vi "Read GMLAN PIDs and DTCs.vi"(8 "error in (no error)":errorcluster, 11 "State Variables":T1={"TCP Refs"={"Connection List"=refnum, "listener ID"=refnum}, "Stop"=refnum, "Top VI"=refnum, "Parameters"={"Name"="", "PID Lookup"=variant, "DID Lookup"=variant, "Section Properties"={"CAN"={"Database File"=path "", "CAN Interface"=enum."CAN0", "Baud Rate"=0, "Diagnostic Protocol"=enum."GMLAN", "Transport Protocol"=enum."ISO TP - Normal Mode", "Transmit ID"=0, "Receive ID"=0, "Transmit Extension"=0, "Receive Extension"=0, "Receive UUDT ID"=0, "Enable Stream"=TRUE, "VW TP Channel ID"=0}, "DPIDs"=[], "DTC descriptor"={"DTC Byte Length"=2, "Status Byte Length"=1, "Add Data Byte Length"=1, "Byte Order"=enum."Motorola"}, "PIDs"=[], "DIDs"=[], "CPIDs"=[]}, "ChanRefs"={"ToVS.PIDs"={"Name"="", "Write to VS Engine FIFO"=refnum, "Pairs"={"Refs"=[], "Values"=[]}}, "ToVS.DIDs"={"Name"="", "Write to VS Engine FIFO"=refnum, "Pairs"={"Refs"=[], "Values"=[]}}, "ToVS.DTCs"={"Name"="", "Write to VS Engine FIFO"=refnum, "Pairs"={"Refs"=[], "Values"=[]}}, "ToVS.DTCCount"={"Name"="", "Write to VS Engine FIFO"=refnum, "Pairs"={"Refs"=[], "Values"=[]}}, "ToVS.Success"={"Name"="", "Write to VS Engine FIFO"=refnum, "Pairs"={"Refs"=[], "Values"=[]}}, "FromVS.CPIDs"={"Name"="", "Read from VS Engine FIFO"=refnum, "Pairs"={"Refs"=[], "Values"=[]}}, "Cmds"={"Name"="", "Write to VS Engine FIFO"=refnum, "Read from VS Engine FIFO"=refnum, "Pairs"={"Chan Refs"=[], "Prev. Values"=[]}}}, "CPID Lookup"=variant, "DPID Lookup"=variant}, "ADCS Connection"={"Diag CAN Handle"=0, "Transport Protocol"=enum."ISO TP - Normal Mode", "Receive Address Extension"=0, "Transmit Address Extension"=0, "Receive CAN Id"=0, "Transmit CAN Id"=0, "Diag CAN Queue"=refnum, "Log Frames ?"=FALSE, "My TP Address"=0, "Other TP Address"=0, "T1"=0, "T2"=0, "T3"=0, "T4"=0, "Tx SN"=0, "Block Size"=0, "Rx SN"=0, "VW TP Initialized?"=FALSE, "Tx block no"=0, "baud rate"=0, "Interface"="", "Channel Diag CAN Handle"=0, "UDP Connection ID"=refnum, "TCP Connection ID"=refnum, "Target IP Addr"=0, "Source Address"=0, "Target Address"=0, "Send Header NACK?"=FALSE, "DLL Handle"=0, "NAD"=0}, "XNET References"={"Database"="", "GMLAN DPID Session"="", "Cluster"=""}, "BufferedCmds"=refnum, "XNETEngine (GMLAN)"=refnum} {"Parameters"."ChanRefs"."Cmds"."Pairs"."Chan Refs" format="%.0x"; "Parameters"."ChanRefs"."ToVS.Success"."Pairs"."Refs" format="%.0x"; "Parameters"."ChanRefs"."ToVS.DTCCount"."Pairs"."Refs" format="%.0x"; "Parameters"."ChanRefs"."ToVS.DTCs"."Pairs"."Refs" format="%.0x"; "Parameters"."ChanRefs"."ToVS.PIDs"."Pairs"."Refs" format="%.0x"; "Parameters"."ChanRefs"."ToVS.DIDs"."Pairs"."Refs" format="%.0x"; "Parameters"."Section Properties"."CPIDs"."Signals"."Byte Order" items=["Little Endian", "Big Endian"]; "Parameters"."Section Properties"."CPIDs"."Signals"."Data Type" items=["Signed", "Unsigned", "IEEE Float"]; "Parameters"."Section Properties"."DIDs"."Signals"."Byte Order" items=["Little Endian", "Big Endian"]; "Parameters"."Section Properties"."DIDs"."Signals"."Data Type" items=["Signed", "Unsigned", "IEEE Float"]; "Parameters"."Section Properties"."CAN"."VW TP Channel ID" format="%.0x"; "Parameters"."Section Properties"."CAN"."Receive UUDT ID" format="%.0x"; "Parameters"."Section Properties"."CAN"."Receive Extension" format="%.0x"; "Parameters"."Section Properties"."CAN"."Transmit Extension" format="%.0x"; "Parameters"."Section Properties"."CAN"."Receive ID" format="%.0x"; "Parameters"."Section Properties"."CAN"."Transmit ID" format="%.0x"; "Parameters"."Section Properties"."PIDs"."Signals"."Byte Order" items=["Little Endian", "Big Endian"]; "Parameters"."Section Properties"."PIDs"."Signals"."Data Type" items=["Signed", "Unsigned", "IEEE Float"]}) -> (0 "error out":errorcluster)   [LabVIEW 2013, in "Diagnostics Addon Engine.lvlib"]
uses:
  Diagnostics Addon Engine.lvlib
  State Variables.ctl
  TCP Refs.ctl
  STM/STM Lookup Table Ref.ctl
  Stop FG/Stop Global Ref.ctl
  Main Configuration.ctl
  Section Properties.ctl
  Shared/CAN Configuration.ctl
  Shared/CAN Interface.ctl
  Shared/Diagnostic Protocols.ctl
  Shared/Transport Protocols.ctl
  Shared/DPID Parameters.ctl
  Shared/DPID Periodic Rate.ctl
  <vilib>/Automotive Diagnostic Command Set/Diagnostic Protocols.llb/DTC Descriptor.ctl
  Shared/DIDPID Parameters.ctl
  Shared/DIDPID Signal Parameters.ctl
  VS Data Channels.ctl
  Inline Async API/Controls/Write To VS Engine.ctl
  <vilib>/NI Veristand/Custom Device API/Data Reference.ctl
  Inline Async API/Controls/Read From VS Engine.ctl
  <vilib>/NI Veristand/Custom Device API/Block Data Reference.ctl
  Inline Async API/Controls/ReadWrite Data.ctl
  <vilib>/Automotive Diagnostic Command Set/Diagnostic Transport.llb/Diag Reference.ctl
  <vilib>/Automotive Diagnostic Command Set/Diagnostic Transport.llb/Transport Protocol Selector.ctl
  <vilib>/Automotive Diagnostic Command Set/Diagnostic Transport.llb/Diag CAN Frame Log.ctl
  XNET References.ctl
  <vilib>/NI/AMC/Message Queue.ctl
  <vilib>/NI/AMC/Message.ctl
  <vilib>/NI/Tools/Keyed Array/KeyedArray.ctl
  Stop FG/Stop Global Commands.ctl
  Change DTC Count Cluster.ctl
  Shared/DTC and Timestamp Cluster.ctl
  <vilib>/xnet/xnet.llb/XNET Frame CAN.ctl
  <vilib>/xnet/xnet.llb/XNET Frame Type CAN.ctl
  PID Data.ctl
  Datatable Lookup Positions.ctl
  DPID Lookup Cluster.ctl
  DPID Lookup PID Information.ctl
  <vilib>/NI/AMC/Create Single Message.vi
  <vilib>/NI/AMC/Update Message Routing Info.vi
  GMLAN/Utilities/Convert Raw Data to DTCs.vi
  <vilib>/NI/AMC/Read Termination Message.vi
  Shared/GUID Lookup.vi
  <vilib>/NI/AMC/Globals.vi
  <vilib>/xnet/xnet.llb/XNET Convert (Frame Raw to Signal).vi
  <vilib>/xnet/xnet.llb/XNET Read (Frame CAN).vi
  <vilib>/Automotive Diagnostic Command Set/Diagnostic Protocols.llb/Convert to Phys.vi
  <vilib>/NI/AMC/Send Message.vi
  Stop FG/Stop FG.lvlib
  Error Handling API/Error Handling API.lvlib
  Shared/Diagnostics Addon Shared.lvlib
  <vilib>/NI Veristand/Custom Device Tools/Custom Device Utility Library/Custom Device Utility Library.lvlib
  <vilib>/NI/AMC/AMC.lvlib
  GMLAN/GMLAN.lvlib
  <vilib>/NI Veristand/Custom Device API/Custom Device API.lvlib
  <vilib>/NI/Tools/Keyed Array/Tools_KeyedArray.lvlib
  <vilib>/addons/Automotive Diagnostic Command Set/NI_Automotive Diagnostic Command Set.lvlib
  Inline Async API/Inline Async API.lvlib
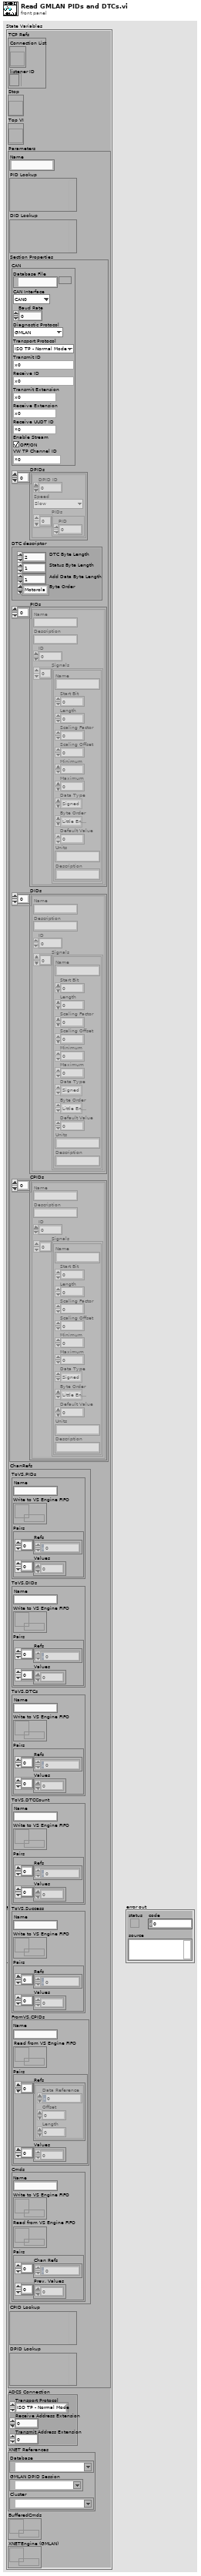
[diagram p1: front panel]
types:
  T1 = typedef "Diagnostics Addon Engine.lvlib/State Variables.ctl" = cluster{"TCP Refs":T2, "Stop":T4, "Top VI":refnum<vi>, "Parameters":T5, "ADCS Connection":T22, "XNET References":T24, "BufferedCmds":T25, "XNETEngine (GMLAN)":T25}
  T2 = typedef "Diagnostics Addon Engine.lvlib/TCP Refs.ctl" = cluster{"Connection List":T3, "listener ID":refnum<k5>}
  T3 = typedef "Diagnostics Addon Engine.lvlib/STM Lookup Table Ref.ctl" = refnum<vi>
  T4 = typedef "Diagnostics Addon Engine.lvlib/Stop FG.lvlib/Stop Global Ref.ctl" = refnum<vi>
  T5 = typedef "Diagnostics Addon Engine.lvlib/Main Configuration.ctl" = cluster{"Name":string, "PID Lookup":variant, "DID Lookup":variant, "Section Properties":T6, "ChanRefs":T16, "CPID Lookup":variant, "DPID Lookup":variant}
  T6 = typedef "Diagnostics Addon Engine.lvlib/Section Properties.ctl" = cluster{"CAN":T7, "DPIDs":T11[], "DTC descriptor":T13, "PIDs":T14[], "DIDs":T14[], "CPIDs":T14[]}
  T7 = typedef "Diagnostics Addon Shared.lvlib/CAN Configuration.ctl" = cluster{"Database File":path, "CAN Interface":T8, "Baud Rate":u32, "Diagnostic Protocol":T9, "Transport Protocol":T10, "Transmit ID":u32, "Receive ID":u32, "Transmit Extension":u8, "Receive Extension":u8, "Receive UUDT ID":u32, "Enable Stream":bool, "VW TP Channel ID":u32}
  T8 = typedef "Diagnostics Addon Shared.lvlib/CAN Interface.ctl" = enum16{"CAN0", "CAN1", "CAN2", "CAN3", "CAN4", "CAN5", "CAN6", "CAN7", "CAN8", "CAN9", "CAN10", "CAN11", "CAN12", "CAN13", "CAN14", "CAN15", "CAN16", "CAN17", "CAN18", "CAN19", "CAN20", "CAN21", "CAN22", "CAN23", "CAN24", "CAN25", "CAN26", "CAN27", "CAN28", "CAN29", "CAN30", "CAN31", "CAN32", "CAN33", "CAN34", "CAN35", "CAN36", "CAN37", "CAN38", "CAN39", "CAN40", "CAN41", "CAN42", "CAN43", "CAN44", "CAN45", "CAN46", "CAN47", "CAN48", "CAN49", "CAN50", "CAN51", "CAN52", "CAN53", "CAN54", "CAN55", "CAN56", "CAN57", "CAN58", "CAN59", "CAN60", "CAN61", "CAN62", "CAN63", "CAN 256 (Virtual)", "CAN 257 (Virtual)"}
  T9 = typedef "Diagnostics Addon Shared.lvlib/Diagnostic Protocols.ctl" = enum16{"GMLAN", "KWP-2000", "UDS"}
  T10 = typedef "Diagnostics Addon Shared.lvlib/Transport Protocols.ctl" = enum16{"ISO TP - Normal Mode", "ISO TP - Mixed Mode", "VW TP 2.0", "Diagnostics on IP"}
  T11 = typedef "Diagnostics Addon Shared.lvlib/DPID Parameters.ctl" = cluster{"DPID ID":u8, "Speed":T12, "PIDs":u16[]}
  T12 = typedef "Diagnostics Addon Shared.lvlib/DPID Periodic Rate.ctl" = enum16{"Slow", "Medium", "Fast"}
  T13 = typedef "DTC Descriptor.ctl" = cluster{"DTC Byte Length":i32, "Status Byte Length":i32, "Add Data Byte Length":i32, "Byte Order":enum16{"Motorola", "Intel"}}
  T14 = typedef "Diagnostics Addon Shared.lvlib/DIDPID Parameters.ctl" = cluster{"Name":string, "Description":string, "ID":u16, "Signals":T15[]}
  T15 = typedef "Diagnostics Addon Shared.lvlib/DIDPID Signal Parameters.ctl" = cluster{"Name":string, "Start Bit":u8, "Length":u8, "Scaling Factor":dbl, "Scaling Offset":dbl, "Minimum":dbl, "Maximum":dbl, "Data Type":u32, "Byte Order":u32, "Default Value":dbl, "Units":string, "Description":string}
  T16 = typedef "Diagnostics Addon Engine.lvlib/VS Data Channels.ctl" = cluster{"ToVS.PIDs":T17, "ToVS.DIDs":T17, "ToVS.DTCs":T17, "ToVS.DTCCount":T17, "ToVS.Success":T17, "FromVS.CPIDs":T19, "Cmds":T21}
  T17 = typedef "Diagnostics Addon Engine.lvlib/Inline Async API.lvlib/Write To VS Engine.ctl" = cluster{"Name":string, "Write to VS Engine FIFO":refnum<k33>, "Pairs":cluster{"Refs":T18[], "Values":dbl[]}}
  T18 = typedef "Custom Device API.lvlib/Data Reference.ctl" = i32
  T19 = typedef "Diagnostics Addon Engine.lvlib/Inline Async API.lvlib/Read From VS Engine.ctl" = cluster{"Name":string, "Read from VS Engine FIFO":refnum<k33>, "Pairs":cluster{"Refs":T20[], "Values":dbl[]}}
  T20 = typedef "Custom Device API.lvlib/Block Data Reference.ctl" = cluster{"Data Reference":T18, "Offset":i32, "Length":i32}
  T21 = typedef "Diagnostics Addon Engine.lvlib/Inline Async API.lvlib/ReadWrite Data.ctl" = cluster{"Name":string, "Write to VS Engine FIFO":refnum<k33>, "Read from VS Engine FIFO":refnum<k33>, "Pairs":cluster{"Chan Refs":T18[], "Prev. Values":dbl[]}}
  T22 = typedef "NI_Automotive Diagnostic Command Set.lvlib/Diag Reference.ctl" = cluster{"Diag CAN Handle":u32, "Transport Protocol":T23, "Receive Address Extension":u8, "Transmit Address Extension":u8, "Receive CAN Id":u32, "Transmit CAN Id":u32, "Diag CAN Queue":refnum<queue>, "Log Frames ?":bool, "My TP Address":u8, "Other TP Address":u8, "T1":u16, "T2":u16, "T3":u16, "T4":u16, "Tx SN":u8, "Block Size":u8, "Rx SN":u8, "VW TP Initialized?":bool, "Tx block no":u8, "baud rate":u32, "Interface":string, "Channel Diag CAN Handle":u32, "UDP Connection ID":refnum<k16>, "TCP Connection ID":refnum<k5>, "Target IP Addr":u32, "Source Address":u16, "Target Address":u16, "Send Header NACK?":bool, "DLL Handle":u32, "NAD":u8}
  T23 = typedef "NI_Automotive Diagnostic Command Set.lvlib/Transport Protocol Selector.ctl" = enum16{"ISO TP - Normal Mode", "ISO TP - Mixed Mode", "VW TP 2.0", "Diagnostics on IP", "ISO TP LIN"}
  T24 = typedef "Diagnostics Addon Engine.lvlib/XNET References.ctl" = cluster{"Database":refnum<k21>, "GMLAN DPID Session":refnum<k21>, "Cluster":refnum<k21>}
  T25 = typedef "AMC.lvlib/Message Queue.ctl" = refnum<queue>
  T26 = typedef "Diagnostics Addon Shared.lvlib/DTC and Timestamp Cluster.ctl" = cluster{"Timestamp":dbl, "DTC":dbl, "Status":dbl, "Add Data":dbl}
  T27 = typedef "Diagnostics Addon Engine.lvlib/Change DTC Count Cluster.ctl" = cluster{"DTCCountChange?":bool, "Timestamp":timestamp}
  T28 = typedef "XNET Frame CAN.ctl" = cluster{"timestamp":timestamp, "payload":u8[], "identifier":u32, "type":T29, "extended?":bool, "echo?":bool}
  T29 = typedef "XNET Frame Type CAN.ctl" = u8
  T30 = cluster{"Change DTC Count Cluster":T27, "Previous DTCs":T26[], "Prev DTC Frames":T28[]}
  T31 = typedef "Diagnostics Addon Engine.lvlib/Stop FG.lvlib/Stop Global Commands.ctl" = enum16{"Write", "Read", "Reset"}
  T32 = typedef "Diagnostics Addon Engine.lvlib/PID Data.ctl" = cluster{"ID":u16, "Raw Frame":u8[]}
  T33 = typedef "Diagnostics Addon Engine.lvlib/Datatable Lookup Positions.ctl" = cluster{"Offset":i32, "Length":i32}
  T34 = typedef "Diagnostics Addon Engine.lvlib/DPID Lookup Cluster.ctl" = cluster{"PID Info":T35, "Datatable Lookup":T33, "Conversion":refnum<k21>}
  T35 = typedef "Diagnostics Addon Engine.lvlib/DPID Lookup PID Information.ctl" = cluster{"PID":u16, "Frame Length":u8}
  T36 = typedef "Diagnostic Trouble Code.ctl" = cluster{"DTC":u32, "Status":u32, "Add Data":u32}
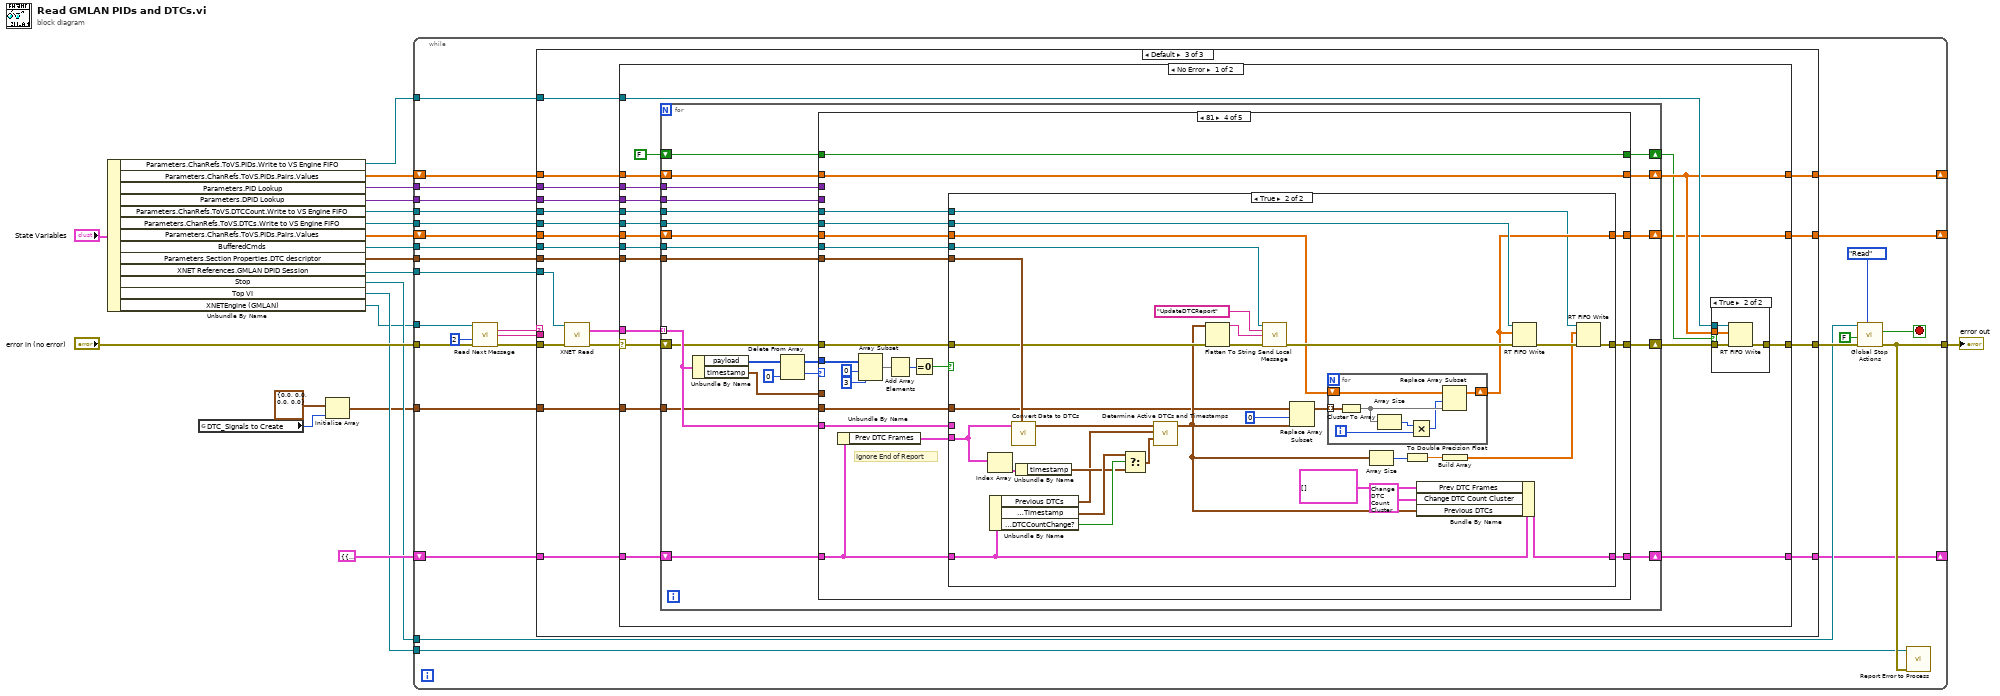
[diagram p0: block diagram]
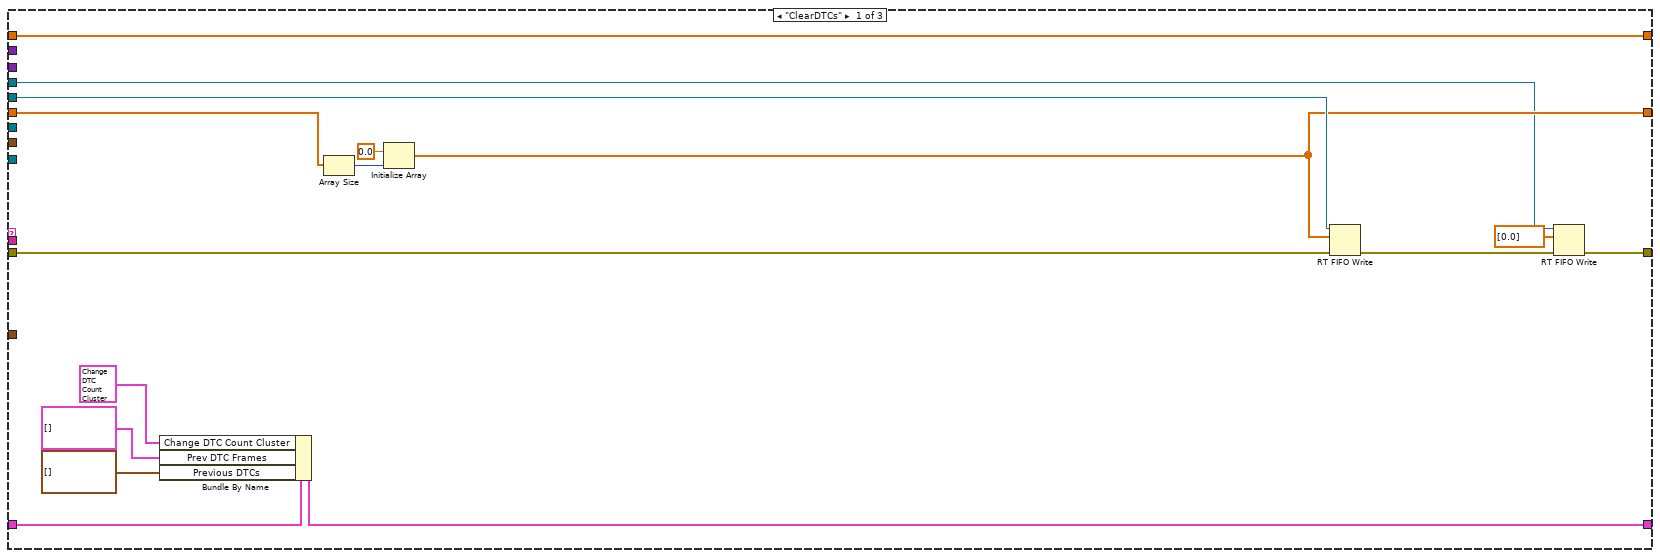
[diagram p2: hidden frame]
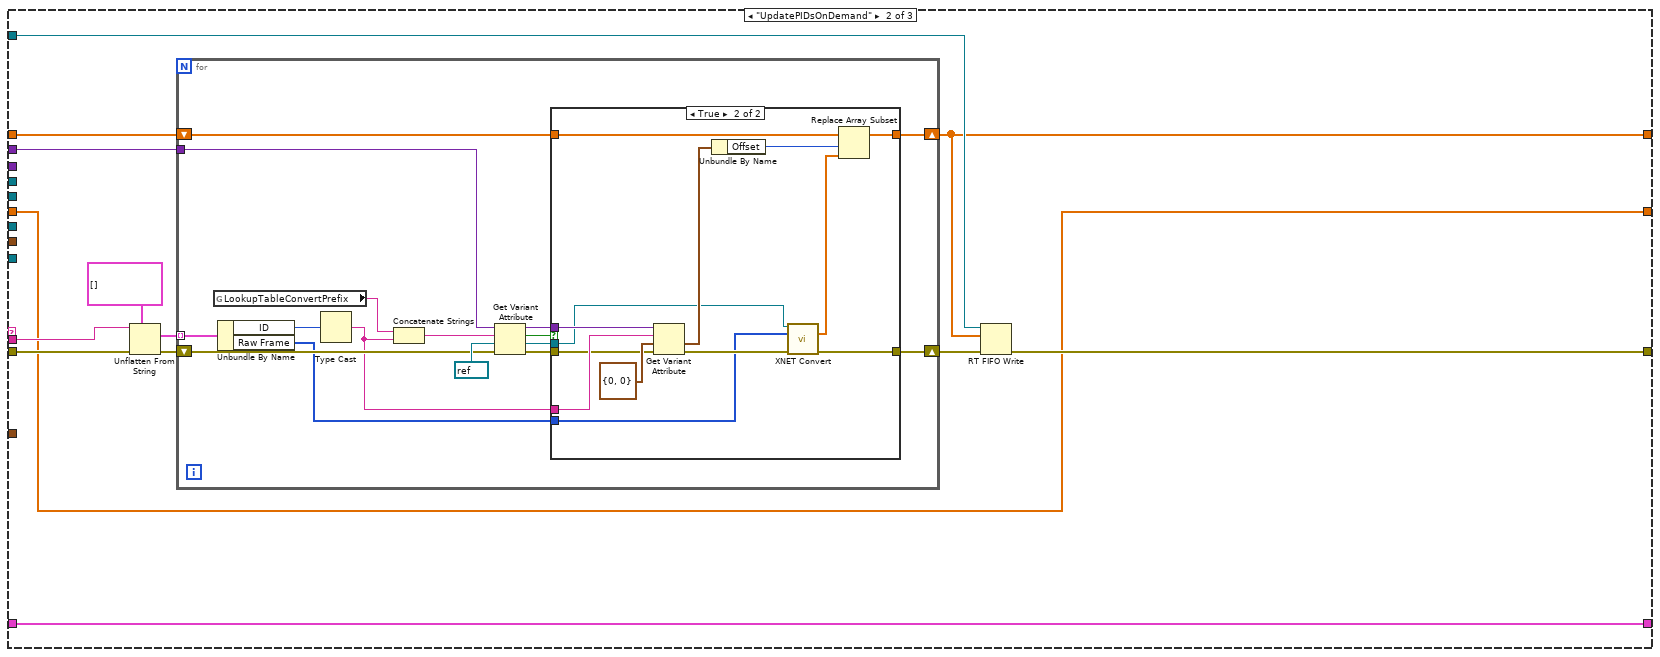
[diagram p3: hidden frame]
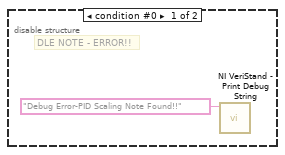
[diagram p5: hidden frame]
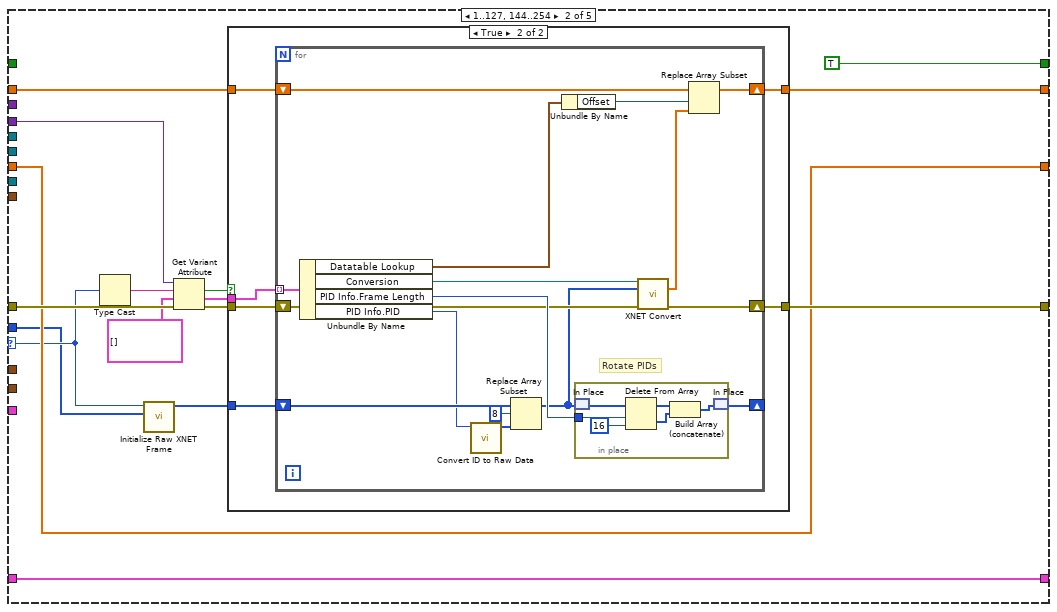
[diagram p7: hidden frame]
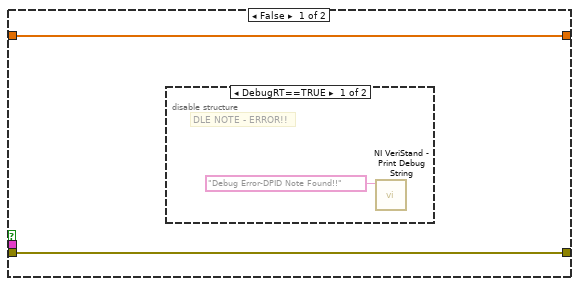
[diagram p8: hidden frame]
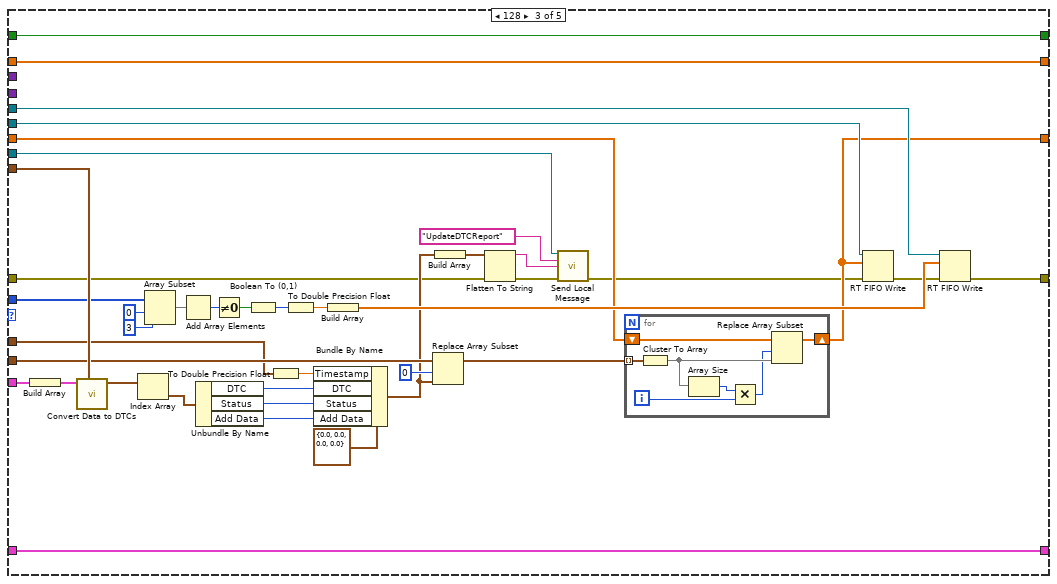
[diagram p10: hidden frame]
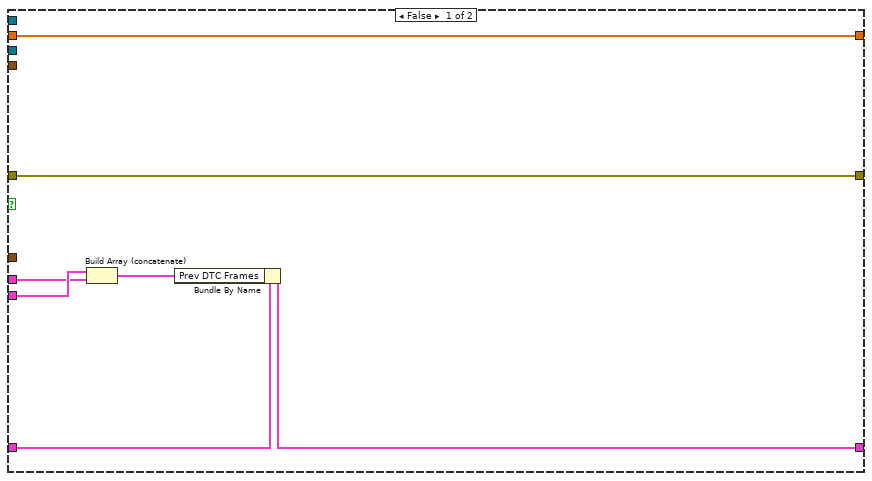
[diagram p11: hidden frame]
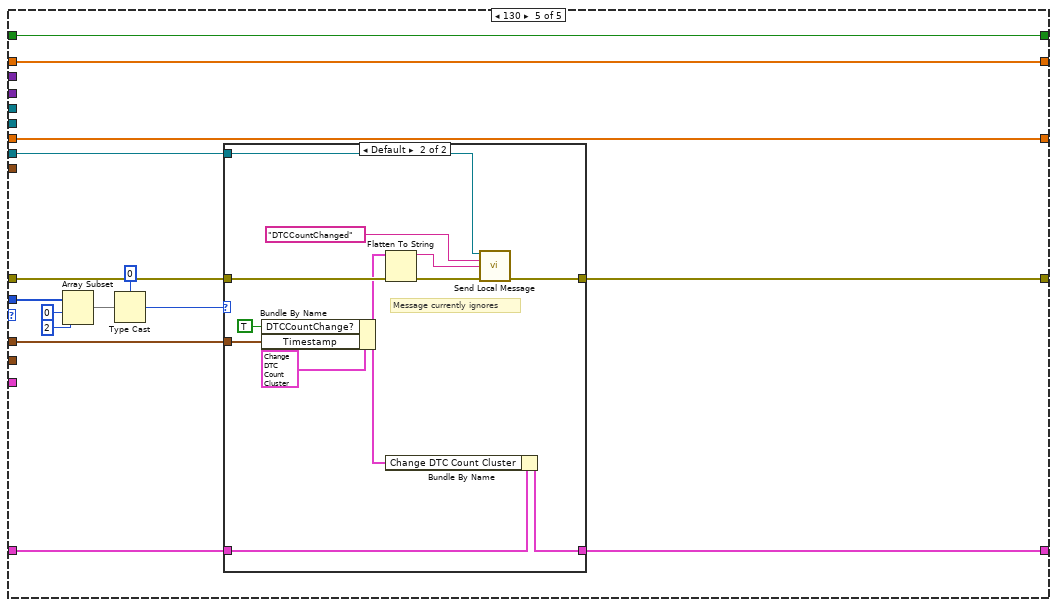
[diagram p12: hidden frame]
diagram:
  n1 = Unbundle By Name("State Variables") -> ("Parameters.ChanRefs.ToVS.PIDs.Write to VS Engine FIFO"=w12:refnum<k33>, "Parameters.ChanRefs.ToVS.PIDs.Pairs.Values"=w8:dbl[], "Parameters.PID Lookup"=w11:variant, "Parameters.DPID Lookup"=w2:variant, "Parameters.ChanRefs.ToVS.DTCCount.Write to VS Engine FIFO"=w6:refnum<k33>, "Parameters.ChanRefs.ToVS.DTCs.Write to VS Engine FIFO"=w17:refnum<k33>, "Parameters.ChanRefs.ToVS.PIDs.Pairs.Values"=w18:dbl[], "BufferedCmds"=w16:T25, "Parameters.Section Properties.DTC descriptor"=w7:T13, "XNET References.GMLAN DPID Session"=w10:refnum<k21>, "Stop"=w13:T4, "Top VI"=w14:refnum<vi>, "XNETEngine (GMLAN)"=w1:T25)
  n2 = global read "GUID Lookup.vi" "DTC_Signals to Create"() -> (w4:i32)
  n3 = Initialize Array(T26 {"Timestamp"=0.0, "DTC"=0.0, "Status"=0.0, "Add Data"=0.0} ("Diagnostic Trouble Code"), w4) -> (w3:T26[])
  n4 = while {
    tunnel: "error in (no error)" -> [w33]
    tunnel: [w45] -> w9
    shift-right: [w40] -> _
    shift-left: w8 -> [w41]
    tunnel: w7 -> [w43]
    tunnel: w10 -> [w42]
    tunnel: w11 -> [w39]
    tunnel: w12 -> [w38]
    tunnel: w16 -> [w37]
    tunnel: w13 -> [w36]
    tunnel: w14 -> [w35]
    tunnel: w1 -> [w25]
    shift-right: [w29] -> _
    shift-left: T30 {"Change DTC Count Cluster"={"DTCCountChange?"=FALSE, "Timestamp"=timestamp(0 s since 1904-01-01)}, "Previous DTCs"=[], "Prev DTC Frames"=[]} -> [w30]
    tunnel: w17 -> [w28]
    shift-right: [w26] -> _
    shift-left: w18 -> [w27]
    tunnel: w6 -> [w24]
    tunnel: w3 -> [w23]
    tunnel: w2 -> [w22]
    stop <- w46 stop-if-true
    n5 = call <vilib>:"Read Next Message.vi"("message queue in"=w25, "timeout (1 ms)"=2 ("timeout (1ms)"), "error in"=w33) -> ("message name"=w31:string, "message value"=w21:string, "error out"=w32:errorcluster)  [unwired: 5 in, 5 out]
    n6 = case shown="Default" w31 {
      tunnel: [w50 w70 w126] -> w44
      tunnel: w43 -> [_ _ w125]
      tunnel: w32 -> [w57 w77 w124]
      tunnel: w42 -> [_ _ w123]
      tunnel: w41 -> [w64 w73 w122]
      tunnel: [w64 w69 w121] -> w40
      tunnel: w39 -> [_ w67 w120]
      tunnel: w38 -> [_ w71 w119]
      tunnel: w37 -> [_ _ w118]
      tunnel: w30 -> [w63 w65 w117]
      tunnel: [w62 w65 w116] -> w29
      tunnel: w28 -> [w58 _ w115]
      tunnel: w27 -> [w54 w66 w114]
      tunnel: [w53 w66 w113] -> w26
      tunnel: w24 -> [w52 _ w112]
      tunnel: w23 -> [_ _ w111]
      tunnel: w22 -> [_ _ w110]
      tunnel: w21 -> [_ w76 _]
      frame "ClearDTCs" {
        n7 = Bundle By Name(cluster=w63, "Change DTC Count Cluster"=T27 {"DTCCountChange?"=FALSE, "Timestamp"=timestamp(0 s since 1904-01-01)}, "Prev DTC Frames"=T28[] [] ("Previous DTC Frames"), "Previous DTCs"=T26[] []) -> (w62:T30)
        n8 = Array Size(array=w54) -> (size(s)=w56:i32)
        n9 = Initialize Array(0.0 ("element"), w56) -> (w53:dbl[])
        n10 = RT FIFO Write(0:w58, 1:w53, 3:w57) -> (11:w51:errorcluster)  [unwired: 2 in, 3 out]
        n11 = RT FIFO Write(0:w52, 1:dbl[] [0.0] ("element"), 3:w51) -> (11:w50:errorcluster)  [unwired: 2 in, 3 out]
      }
      frame "UpdatePIDsOnDemand" {
        n12 = Unflatten From String(type=T32[] [], binary string=w76, error in (no error)=w77) -> (value=w68:T32[], error out=w74:errorcluster)  [unwired: 2 in, 1 out]
        n13 = for {
          shift-right: [w85] -> w72
          shift-left: w74 -> [w86]
          shift-right: [w83] -> w69
          shift-left: w73 -> [w84]
          tunnel: w68 -> [w82] mode=indexing
          tunnel: w67 -> [w80]
          n14 = global read "GUID Lookup.vi" "LookupTableConvertPrefix"() -> (w93:string)
          n15 = Unbundle By Name(w82) -> ("ID"=w81:u16, "Raw Frame"=w78:u8[])
          n16 = Type Cast(x=w81) -> (*(type *) &x=w79:string)  [unwired: 1 in]
          n17 = Concatenate Strings(w93, w79) -> (w92:string)
          n18 = Get Variant Attribute(Variant=w80, name=w92, default value (empty Variant)=refnum<k21> refnum ("DID Conversion"), error in=w86) -> (duplicate Variant=w88:variant, found=w87:bool, value=w89:refnum<k21>, error out=w90:errorcluster)
          n19 = case shown="True" w87 {
            tunnel: [w95 w102] -> w85
            tunnel: w84 -> [w94 w98]
            tunnel: [w94 w107] -> w83
            tunnel: w90 -> [w95 w104]
            tunnel: w89 -> [_ w101]
            tunnel: w79 -> [_ w106]
            tunnel: w88 -> [_ w105]
            tunnel: w78 -> [_ w99]
            frame False {
              n20 = disable-structure shown="Default" {
                frame condition #0 {
                  # "DLE NOTE - ERROR!!"
                  n21 = call <vilib>:"NI VeriStand - Print Debug String.vi"("Message"="Debug Error-PID Scaling Note Found!!" ("Debug String")) -> ()  [unwired: 10 in, 1 out]
                }
                frame condition #1 (active) {
                }
              }
            }
            frame True {
              n22 = Get Variant Attribute(Variant=w105, name=w106, default value (empty Variant)=T33 {"Offset"=0, "Length"=0} ("cluster"), error in=w104) -> (value=w108:T33, error out=w103:errorcluster)  [unwired: 2 out]
              n23 = Unbundle By Name(w108) -> ("Offset"=w97:i32)
              n24 = call-poly <vilib>:"XNET Convert.vi"("session in"=w101, "frame data"=w99, "error in (no error)"=w103) -> ("signal data"=w100:dbl[], "error out"=w102:errorcluster)  [unwired: 10 in, 1 out]
              n25 = Replace Array Subset(array=w98, new element=w100, index=w97) -> (w107:dbl[])
            }
          }
        }
        n26 = RT FIFO Write(0:w71, 1:w69, 3:w72) -> (11:w70:errorcluster)  [unwired: 2 in, 3 out]
      }
      frame Default {
        n27 = call-poly <vilib>:"XNET Read.vi"("session in"=w123, "error in (no error)"=w124) -> ("data"=w127:T28[], "error out"=w128:errorcluster)  [unwired: 10 in, 2 out]
        n28 = case shown="No Error" w128 {
          selector: w128 -> [w147 w375]
          tunnel: w127 -> [w148 _]
          tunnel: [w142 w375] -> w126
          tunnel: w125 -> [w145 _]
          tunnel: w122 -> [w144 w374]
          tunnel: [w140 w374] -> w121
          tunnel: w120 -> [w143 _]
          tunnel: w119 -> [w141 _]
          tunnel: w118 -> [w139 _]
          tunnel: w117 -> [w136 w373]
          tunnel: [w135 w373] -> w116
          tunnel: w115 -> [w134 _]
          tunnel: w114 -> [w133 w372]
          tunnel: [w132 w372] -> w113
          tunnel: w112 -> [w131 _]
          tunnel: w111 -> [w130 _]
          tunnel: w110 -> [w129 _]
          frame No Error {
            n29 = for {
              tunnel: w148 -> [w171] mode=indexing
              shift-right: [w149] -> w146
              shift-left: w147 -> [w150]
              tunnel: w145 -> [w170]
              shift-right: [w169] -> w140
              shift-left: w144 -> [w168]
              tunnel: w143 -> [w167]
              tunnel: w139 -> [w166]
              shift-right: [w163] -> w137
              shift-left: FALSE -> [w164]
              shift-right: [w162] -> w135
              shift-left: w136 -> [w161]
              tunnel: w134 -> [w160]
              shift-right: [w158] -> w132
              shift-left: w133 -> [w159]
              tunnel: w131 -> [w157]
              tunnel: w130 -> [w156]
              tunnel: w129 -> [w155]
              n30 = Unbundle By Name(w171) -> ("payload"=w153:u8[], "timestamp"=w165:timestamp)
              n31 = Delete From Array(array=w153, index=0) -> (deleted portion=w151:u8, array with subset deleted=w152:u8[])  [unwired: 1 in]
              n32 = case shown="81" w151 {
                selector: w151 -> [_ w178 _ _ _]
                tunnel: w152 -> [_ w177 w252 w291 w350]
                tunnel: w171 -> [_ _ w263 w272 _]
                tunnel: [w176 w192 w224 w282 w346] -> w149
                tunnel: w150 -> [w176 w187 w226 w283 w345]
                tunnel: w170 -> [_ _ w261 w284 _]
                tunnel: [w175 w190 w260 w286 w347] -> w169
                tunnel: w168 -> [w175 w191 w260 w286 w347]
                tunnel: w167 -> [_ _ _ _ _]
                tunnel: w166 -> [_ _ w229 w275 w338]
                tunnel: w165 -> [_ _ w238 _ w344]
                tunnel: w164 -> [w174 _ w259 w279 w343]
                tunnel: [w174 TRUE w259 w279 w343] -> w163
                tunnel: [w173 w188 w258 w281 w340] -> w162
                tunnel: w161 -> [w173 w188 w258 w280 w341]
                tunnel: w160 -> [_ _ w234 w278 _]
                tunnel: w159 -> [w172 w185 w236 w277 w342]
                tunnel: [w172 w185 w233 w276 w342] -> w158
                tunnel: w157 -> [_ _ w257 w274 _]
                tunnel: w156 -> [_ _ w245 w271 _]
                tunnel: w155 -> [_ w180 _ _ _]
                frame Default {
                }
                frame 1..127, 144..254 {
                  n33 = Type Cast(x=w178) -> (*(type *) &x=w183:string)  [unwired: 1 in]
                  n34 = call "Initialize Raw XNET Frame.vi"("Data"=w177, "identifier"=w178) -> ("Raw Frame"=w179:u8[])  [unwired: 9 in]
                  n35 = Get Variant Attribute(Variant=w180, name=w183, default value (empty Variant)=T34[] [], error in=w187) -> (found=w181:bool, value=w184:T34[], error out=w186:errorcluster)  [unwired: 1 out]
                  n36 = case shown="True" w181 {
                    tunnel: [w194 w201] -> w192
                    tunnel: w191 -> [w193 w200]
                    tunnel: [w193 w199] -> w190
                    tunnel: w186 -> [w194 w198]
                    tunnel: w184 -> [_ w197]
                    tunnel: w179 -> [_ w196]
                    frame False {
                      n37 = disable-structure shown="DebugRT==TRUE" {
                        frame condition #0 {
                          # "DLE NOTE - ERROR!!"
                          n38 = call <vilib>:"NI VeriStand - Print Debug String.vi"("Message"="Debug Error-DPID Note Found!!" ("Debug String")) -> ()  [unwired: 10 in, 1 out]
                        }
                        frame condition #1 (active) {
                        }
                      }
                    }
                    frame True {
                      n39 = for {
                        shift-right: [w215] -> w199
                        shift-left: w200 -> [w216]
                        shift-right: [w217] -> w201
                        shift-left: w198 -> [w207]
                        tunnel: w197 -> [w214] mode=indexing
                        shift-right: [w211] -> _
                        shift-left: w196 -> [w212]
                        # "Rotate PIDs"
                        n40 = Unbundle By Name(w214) -> ("Datatable Lookup"=w206:T33, "Conversion"=w210:refnum<k21>, "PID Info.Frame Length"=w213:u8, "PID Info.PID"=w205:u16)
                        n41 = call "Convert ID to Raw Data.vi"("identifier"=w205) -> ("Data"=w203:u8[])  [unwired: 10 in]
                        n42 = Replace Array Subset(array=w212, new element=w203, index=8) -> (w204:u8[])
                        n43 = Unbundle By Name(w206) -> ("Offset"=w209:i32)
                        n44 = in-place {
                          in-place-border: w213 -> [w222]
                          n45 = in-place-match #1(w204) -> (w221:u8[])
                          n46 = Delete From Array(array=w221, length=w222, index=16 ("length")) -> (deleted portion=w219:u8[], array with subset deleted=w220:u8[])
                          n47 = Build Array (concatenate)(w220, w219) -> (w218:u8[])
                          n48 = in-place-match #1(w218) -> (w211:u8[])
                        }
                        n49 = call-poly <vilib>:"XNET Convert.vi"("session in"=w210, "frame data"=w204, "error in (no error)"=w207) -> ("signal data"=w208:dbl[], "error out"=w217:errorcluster)  [unwired: 10 in, 1 out]
                        n50 = Replace Array Subset(array=w216, new element=w208, index=w209) -> (w215:dbl[])
                      }
                    }
                  }
                }
                frame 128 {
                  n51 = Build Array(w263) -> (w262:T28[])
                  n52 = call "Convert Data to DTCs.vi"("DTC descriptor"=w261, "All DTCs"=w262) -> ("DTCs"=w244:T36[])  [unwired: 8 in, 1 out]
                  n53 = Index Array(array=w244) -> (element=w242:T36)  [unwired: 1 in]
                  n54 = Array Subset(array=w252, index=0, length=3) -> (w254:u8[])
                  n55 = Add Array Elements(numeric array=w254) -> (sum=w253:u8)
                  n56 = Unbundle By Name(w242) -> ("DTC"=w239:u32, "Status"=w240:u32, "Add Data"=w241:u32)
                  n57 = Not Equal To 0?(x=w253) -> (x != 0?=w251:bool)
                  n58 = Boolean To (0,1)(Boolean=w251) -> (0, 1=w250:i16)
                  n59 = To Double Precision Float(number=w238) -> (double precision float=w237:dbl)
                  n60 = To Double Precision Float(number=w250) -> (double precision float=w249:dbl)
                  n61 = Bundle By Name(cluster=T26 {"Timestamp"=0.0, "DTC"=0.0, "Status"=0.0, "Add Data"=0.0} ("Diagnostic Trouble Code"), "Timestamp"=w237, "DTC"=w239, "Status"=w240, "Add Data"=w241) -> (w228:T26)
                  n62 = Build Array(w249) -> (w248:dbl[])
                  n63 = Replace Array Subset(array=w245, new element=w228, index=0) -> (w246:T26[])
                  n64 = Build Array(w228) -> (w227:T26[])
                  n65 = Flatten To String(anything=w227, error in (no error)=w226) -> (data string=w230:string, error out=w231:errorcluster)  [unwired: 2 in, 1 out]
                  n66 = call <vilib>:"Send Local Message.vi"("message queue in"=w229, "message name"="UpdateDTCReport" ("Message Name"), "message value"=w230, "error in"=w231) -> ("error out"=w225:errorcluster)  [unwired: 9 in, 2 out]
                  n67 = for {
                    tunnel: w246 -> [w270] mode=indexing
                    shift-right: [w269] -> w233
                    shift-left: w236 -> [w268]
                    i -> [w265]
                    n68 = Cluster To Array(cluster=w270) -> (array=w267:dbl[])
                    n69 = Array Size(array=w267) -> (size(s)=w266:i32)
                    n70 = Multiply(x=w266, y=w265) -> (x*y=w264:i32)
                    n71 = Replace Array Subset(array=w268, new element=w267, index=w264) -> (w269:dbl[])
                  }
                  n72 = RT FIFO Write(0:w234, 1:w233, 3:w225) -> (11:w235:errorcluster)  [unwired: 2 in, 3 out]
                  n73 = RT FIFO Write(0:w257, 1:w248, 3:w235) -> (11:w224:errorcluster)  [unwired: 2 in, 3 out]
                }
                frame 129 {
                  # "Ignore End of Report"
                  n74 = Unbundle By Name(w280) -> ("Prev DTC Frames"=w273:T28[])
                  n75 = Array Subset(array=w291, index=0, length=3) -> (w288:u8[])
                  n76 = Add Array Elements(numeric array=w288) -> (sum=w287:u8)
                  n77 = Equal To 0?(x=w287) -> (x = 0?=w285:bool)
                  n78 = case shown="True" w285 {
                    tunnel: w284 -> [_ w330]
                    tunnel: w275 -> [_ w299]
                    tunnel: w283 -> [w298 w323]
                    tunnel: [w298 w307] -> w282
                    tunnel: w280 -> [w297 w322]
                    tunnel: [w296 w320] -> w281
                    tunnel: w278 -> [_ w316]
                    tunnel: w277 -> [w295 w315]
                    tunnel: [w295 w314] -> w276
                    tunnel: w274 -> [_ w306]
                    tunnel: w273 -> [w294 w302]
                    tunnel: w272 -> [w293 _]
                    tunnel: w271 -> [_ w300]
                    frame False {
                      n79 = Build Array (concatenate)(w294, w293) -> (w292:T28[])
                      n80 = Bundle By Name(cluster=w297, "Prev DTC Frames"=w292) -> (w296:T30)
                    }
                    frame True {
                      n81 = Index Array(array=w302) -> (element=w311:T28)  [unwired: 1 in]
                      n82 = Unbundle By Name(w322) -> ("Previous DTCs"=w309:T26[], "Change DTC Count Cluster.Timestamp"=w318:timestamp, "Change DTC Count Cluster.DTCCountChange?"=w329:bool)
                      n83 = call "Convert Data to DTCs.vi"("DTC descriptor"=w330, "All DTCs"=w302) -> ("DTCs"=w325:T36[])  [unwired: 8 in, 1 out]
                      n84 = Unbundle By Name(w311) -> ("timestamp"=w310:timestamp)
                      n85 = Select(t=w318, s=w329, f=w310) -> (s? t:f=w324:timestamp)
                      n86 = call "Determine Active DTCs and Timestamps.vi"("current Time Stamp"=w324, "Previous Changed DTCs"=w309, "current DTCs"=w325) -> ("Active DTCs"=w301:T26[])  [unwired: 8 in]
                      n87 = Flatten To String(anything=w301, error in (no error)=w323) -> (data string=w326:string, error out=w327:errorcluster)  [unwired: 2 in, 1 out]
                      n88 = call <vilib>:"Send Local Message.vi"("message queue in"=w299, "message name"="UpdateDTCReport" ("Message Name"), "message value"=w326, "error in"=w327) -> ("error out"=w317:errorcluster)  [unwired: 9 in, 2 out]
                      n89 = Replace Array Subset(array=w300, new element=w301, index=0) -> (w312:T26[])
                      n90 = for {
                        tunnel: w312 -> [w337] mode=indexing
                        shift-right: [w336] -> w314
                        shift-left: w315 -> [w335]
                        i -> [w332]
                        n91 = Cluster To Array(cluster=w337) -> (array=w334:dbl[])
                        n92 = Array Size(array=w334) -> (size(s)=w333:i32)
                        n93 = Multiply(x=w333, y=w332) -> (x*y=w331:i32)
                        n94 = Replace Array Subset(array=w335, new element=w334, index=w331) -> (w336:dbl[])
                      }
                      n95 = Array Size(array=w301) -> (size(s)=w305:i32)
                      n96 = To Double Precision Float(number=w305) -> (double precision float=w303:dbl)
                      n97 = Bundle By Name(cluster=w322, "Prev DTC Frames"=T28[] [] ("data"), "Change DTC Count Cluster"=T27 {"DTCCountChange?"=FALSE, "Timestamp"=timestamp(0 s since 1904-01-01)}, "Previous DTCs"=w301) -> (w320:T30)
                      n98 = Build Array(w303) -> (w304:dbl[])
                      n99 = RT FIFO Write(0:w316, 1:w314, 3:w317) -> (11:w308:errorcluster)  [unwired: 2 in, 3 out]
                      n100 = RT FIFO Write(0:w306, 1:w304, 3:w308) -> (11:w307:errorcluster)  [unwired: 2 in, 3 out]
                    }
                  }
                }
                frame 130 {
                  n101 = Array Subset(array=w350, index=0, length=2) -> (w349:u8[])
                  n102 = Type Cast(type=u16 0 ("length"), x=w349) -> (*(type *) &x=w339:u16)
                  n103 = case shown="Default" w339 {
                    tunnel: [w354 w366] -> w346
                    tunnel: w345 -> [w354 w363]
                    tunnel: w344 -> [_ w362]
                    tunnel: w341 -> [w353 w358]
                    tunnel: [w353 w357] -> w340
                    tunnel: w338 -> [_ w355]
                    frame 0 {
                      # "ChangeDTCCount Disabled."
                    }
                    frame Default {
                      # "Message currently ignores"
                      n104 = Bundle By Name(cluster=T27 {"DTCCountChange?"=FALSE, "Timestamp"=timestamp(0 s since 1904-01-01)} ("Cluster"), "DTCCountChange?"=TRUE, "Timestamp"=w362) -> (w359:T27)
                      n105 = Flatten To String(anything=w359, error in (no error)=w363) -> (data string=w365:string, error out=w364:errorcluster)  [unwired: 2 in, 1 out]
                      n106 = Bundle By Name(cluster=w358, "Change DTC Count Cluster"=w359) -> (w357:T30)
                      n107 = call <vilib>:"Send Local Message.vi"("message queue in"=w355, "message name"="DTCCountChanged" ("Message Name"), "message value"=w365, "error in"=w364) -> ("error out"=w366:errorcluster)  [unwired: 9 in, 2 out]
                    }
                  }
                }
              }
            }
            n108 = case shown="True" w137 {
              tunnel: w146 -> [w367 w371]
              tunnel: [w367 w370] -> w142
              tunnel: w141 -> [_ w369]
              tunnel: w140 -> [_ w368]
              frame False {
              }
              frame True {
                n109 = RT FIFO Write(0:w369, 1:w368, 3:w371) -> (11:w370:errorcluster)  [unwired: 2 in, 3 out]
              }
            }
          }
          frame Error {
          }
        }
      }
    }
    n110 = call "Global Stop Actions.vi"("Command"=Stop_Global_Commands."Read", "error in (no error)"=w44, "Stop on Error?"=FALSE, "vi reference"=w36) -> ("error out"=w45:errorcluster, "Latched Stop"=w46:bool)  [unwired: 5 in, 1 out]
    n111 = call "Report Error to Process.vi"("Error"=w45, "This VI"=w35) -> ()  [unwired: 10 in]
  }
  "error out" <- w9
